vi "Read Asynchronous Measurement.vi"   [LabVIEW 2017, in "Keithley 2600 Series.lvlib"]
doc: "Returns the asynchronous measurements."
uses:
  <instrlib>/Keithley 2600 Series/Keithley 2600 Series.lvlib
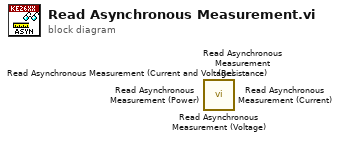
[diagram p0: block diagram]
diagram:
  n1 = call <instrlib>:"Read Asynchronous Measurement (Voltage).vi"() -> ()  [unwired: 9 in, 3 out]
  n2 = call <instrlib>:"Read Asynchronous Measurement (Resistance).vi"() -> ()  [unwired: 9 in, 3 out]
  n3 = call <instrlib>:"Read Asynchronous Measurement (Power).vi"() -> ()  [unwired: 9 in, 3 out]
  n4 = call <instrlib>:"Read Asynchronous Measurement (Current).vi"() -> ()  [unwired: 9 in, 3 out]
  n5 = call <instrlib>:"Read Asynchronous Measurement (Current and Voltage).vi"() -> ()  [unwired: 8 in, 4 out]
